vi "ex_Modify Signals Names.vi"(8 "error in (no error)":errorcluster caption="Fehler (Eingang, kein Fehler)", 10 "Name Modifier":string caption="Namen-Modifizierer", 11 "Array of Waveforms In":waveform(dbl)[](array[waveform]) caption="Signalverlaufs-Array (Eingang)") -> (0 "error out":errorcluster caption="Fehler (Ausgang)", 3 "Array of Waveforms Out":waveform(dbl)[](array[waveform]) caption="Signalverlaufs-Array (Ausgang)")   [LabVIEW 2009]
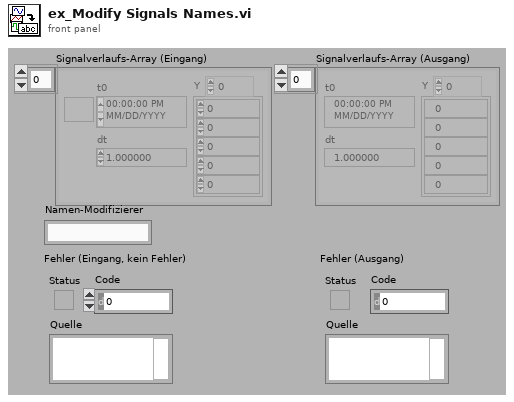
[diagram p1: front panel]
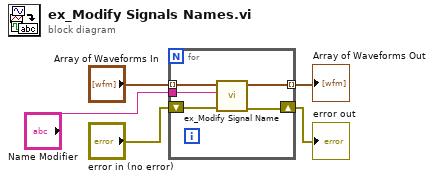
[diagram p0: block diagram]
diagram:
  n1 = for {
    tunnel: "Array of Waveforms In" -> [w10] mode=indexing
    tunnel: [w9] -> w5 mode=indexing
    shift-right: [w8] -> w3
    shift-left: "error in (no error)" -> [w7]
    tunnel: "Name Modifier" -> [w6]
    n2 = call "ex_Modify Signal Name.vi"("error in (no error)"=w7, "Name Modifier"=w6, "waveform in"=w10) -> ("error out"=w8:errorcluster, "waveform out"=w9:waveform(dbl))  [unwired: 7 in]
  }
  "Array of Waveforms Out" <- w5
  "error out" <- w3
